vi "test_timer_stop-point.vi"() -> ()   [LabVIEW 2019]
panel:
  out "time-out":bool
  out "time_status_out":T1 {"total time" format="%.1f"; "run time" format="%.1f"; "pause time" format="%.1f"}
  in  "start":bool
  in  "정지":bool
  in  "target time":dbl=5.0
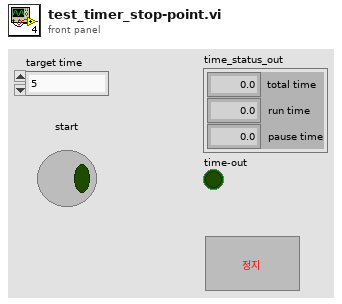
[diagram p1: front panel]
types:
  T1 = cluster{"total time":dbl, "run time":dbl, "pause time":dbl}
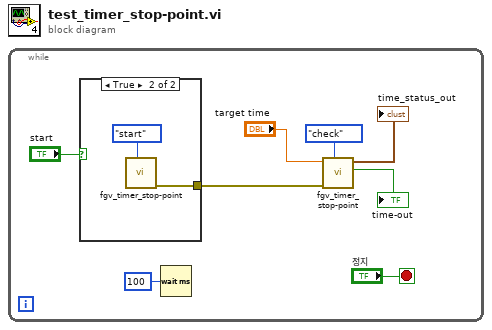
[diagram p0: block diagram]
diagram:
  n1 = while {
    stop <- "정지" stop-if-true
    n2 = case shown="True" "start" {
      tunnel: [_ w9] -> w2
      frame False {
      }
      frame True {
        n3 = call "fgv_timer_stop-point.vi"("cmd"=enum16{"check", "start", "pause"}."start") -> ("error out"=w9:errorcluster)  [unwired: 8 in, 2 out]
      }
    }
    n4 = Wait (ms)(milliseconds to wait=u32 100 ("대기 시간 (ms)")) -> ()  [unwired: 1 out]
    n5 = call "fgv_timer_stop-point.vi"("cmd"=enum16{"check", "start", "pause"}."check", "error in"=w2, "target time"="target time") -> ("time-out"=→"time-out":bool, "time_status_out"=→"time_status_out":T1)  [unwired: 6 in, 1 out]
  }
